vi "main.vi"() -> ()   [LabVIEW 2024]
uses:
  speed.ctl
panel:
  in  "stop":bool
  out "elements in queue":i32
  in  "Enqueue Speed":T1
  in  "Dequeue Speed":T1
  out "EnqueueOut2":dbl(knob) scale=0.0..1.0
  out "EnqueueOut":dbl
  out "dequeueOut2":dbl(knob) scale=0.0..1.0
  out "dequeueOut":dbl
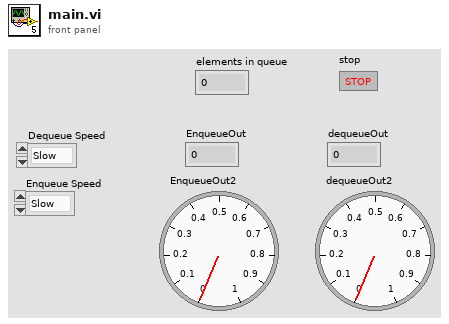
[diagram p1: front panel]
types:
  T1 = typedef "speed.ctl" = enum16{"Slow", "Fast"}
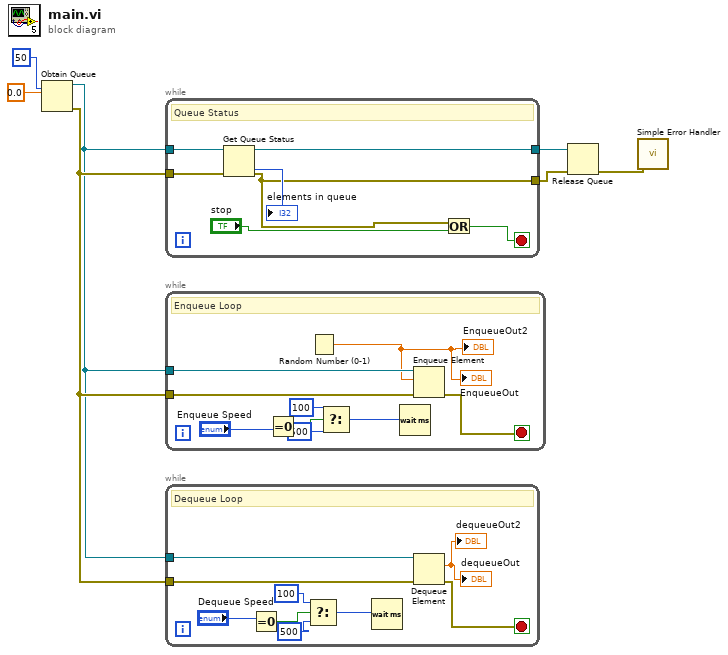
[diagram p0: block diagram]
diagram:
  n1 = Obtain Queue(max queue size (-1, unlimited)=50, element data type=0.0) -> (queue out=w4:refnum<queue>, error out=w5:errorcluster)  [unwired: 3 in, 1 out]
  n2 = while {
    tunnel: w5 -> [w14]
    tunnel: w4 -> [w13]
    tunnel: [w9] -> w3
    tunnel: [w8] -> w2
    stop <- w10 stop-if-true
    # "Queue Status"
    n3 = Get Queue Status(queue=w13, error in (no error)=w14) -> (queue out=w9:refnum<queue>, error out=w8:errorcluster, # elements in queue=→"elements in queue":i32)  [unwired: 1 in, 5 out]
    n4 = Or(x=w8, y="stop") -> (x .or. y?=w10:bool)
  }
  n5 = while {
    tunnel: w5 -> [w22]
    tunnel: w4 -> [w21]
    stop <- w23 stop-if-true
    # "Enqueue Loop"
    n6 = Equal To 0?(x="Enqueue Speed") -> (x = 0?=w18:bool)
    n7 = Random Number (0-1)() -> (number: 0 to 1=w20:dbl)
    "EnqueueOut2" <- w20
    "EnqueueOut" <- w20
    n8 = Select(t=100, s=w18, f=500) -> (s? t:f=w17:i32)
    n9 = Wait (ms)(milliseconds to wait=w17) -> ()  [unwired: 1 out]
    n10 = Enqueue Element(queue=w21, element=w20, error in (no error)=w22) -> (error out=w23:errorcluster)  [unwired: 1 in, 2 out]
  }
  n11 = while {
    tunnel: w5 -> [w31]
    tunnel: w4 -> [w30]
    stop <- w32 stop-if-true
    # "Dequeue Loop"
    n12 = Equal To 0?(x="Dequeue Speed") -> (x = 0?=w27:bool)
    n13 = Select(t=100, s=w27, f=500) -> (s? t:f=w26:i32)
    n14 = Wait (ms)(milliseconds to wait=w26) -> ()  [unwired: 1 out]
    n15 = Dequeue Element(queue=w30, error in (no error)=w31) -> (element=→"dequeueOut2" →"dequeueOut":dbl, error out=w32:errorcluster)  [unwired: 1 in, 2 out]
  }
  n16 = Release Queue(queue=w3, error in (no error)=w2) -> (error out=w1:errorcluster)  [unwired: 1 in, 2 out]
  n17 = call <vilib>:"Simple Error Handler.vi"("error in (no error)"=w1) -> ()  [unwired: 4 in, 5 out]
